vi "basic-lifetime-test.vi"(8 "error in (no error)":errorcluster) -> (0 "error out":errorcluster)   [LabVIEW 2021]
uses:
  <vilib>/addons/_JKI Toolkits/Caraya/classes/Test/Test.lvclass
  src/SMO/SMO.lvclass
  <vilib>/addons/_JKI Toolkits/Caraya/classes/Assert/Assert.lvclass
  src/SMO/Typedefs/SMOState --Enum.ctl
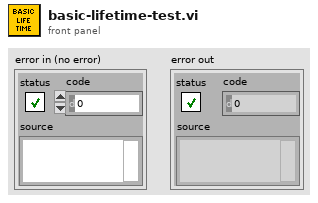
[diagram p1: front panel]
types:
  T1 = typedef "smo.lvlib/SMO.lvclass/SMOState --Enum.ctl" = enum16{"unknown", "Created", "Started", "Stopped"}
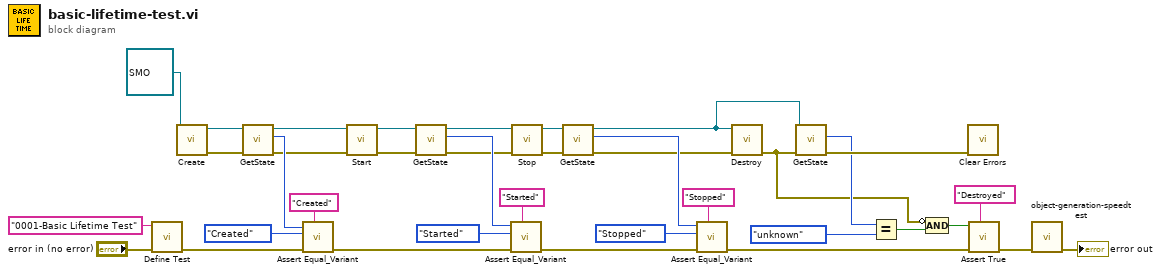
[diagram p0: block diagram]
diagram:
  n1 = call <vilib>:"Define Test.vi"("error in (no error)"="error in (no error)", "Label (VI Title)"="0001-Basic Lifetime Test") -> ("error out"=w33:errorcluster)  [unwired: 9 in]
  n2 = call "Create.vi"("SMO"=refnum<class "SMO.lvclass"> refnum ("Dependency Type")) -> ("error out"=w34:errorcluster, "SMO out"=w36:refnum<class "SMO.lvclass">)  [unwired: 8 in, 1 out]
  n3 = call "GetState.vi"("error in (no error)"=w34, "SMO"=w36) -> ("error out"=w29:errorcluster, "SMO State"=w32:T1, "SMO out"=w35:refnum<class "SMO.lvclass">)  [unwired: 7 in]
  n4 = call <vilib>:"Assert Equal_Variant.vi"("Label"="Created" ("Label (VI Title)"), "error in (no error)"=w33, "Y"=SMOState_--Enum."Created" ("SMO State"), "X"=w32) -> ("error out"=w25:errorcluster)  [unwired: 7 in]
  n5 = call "Start.vi"("error in (no error)"=w29, "SMO"=w35) -> ("error out"=w27:errorcluster, "SMO out"=w28:refnum<class "SMO.lvclass">)  [unwired: 8 in]
  n6 = call "GetState.vi"("error in (no error)"=w27, "SMO"=w28) -> ("error out"=w21:errorcluster, "SMO State"=w23:T1, "SMO out"=w22:refnum<class "SMO.lvclass">)  [unwired: 7 in]
  n7 = call <vilib>:"Assert Equal_Variant.vi"("Label"="Started" ("Label (VI Title)"), "error in (no error)"=w25, "Y"=SMOState_--Enum."Started" ("SMO State"), "X"=w23) -> ("error out"=w15:errorcluster)  [unwired: 7 in]
  n8 = call "Stop.vi"("error in (no error)"=w21, "SMO"=w22) -> ("error out"=w18:errorcluster, "SMO out"=w17:refnum<class "SMO.lvclass">)  [unwired: 8 in]
  n9 = call "GetState.vi"("error in (no error)"=w18, "SMO"=w17) -> ("error out"=w14:errorcluster, "SMO State"=w16:T1, "SMO out"=w13:refnum<class "SMO.lvclass">)  [unwired: 7 in]
  n10 = call <vilib>:"Assert Equal_Variant.vi"("Label"="Stopped" ("Label (VI Title)"), "error in (no error)"=w15, "Y"=SMOState_--Enum."Stopped" ("SMO State"), "X"=w16) -> ("error out"=w6:errorcluster)  [unwired: 7 in]
  n11 = call "Destroy.vi"("error in (no error)"=w14, "SMO"=w13) -> ("error out"=w7:errorcluster)  [unwired: 9 in]
  n12 = call "GetState.vi"("error in (no error)"=w7, "SMO"=w13) -> ("error out"=w11:errorcluster, "SMO State"=w9:T1)  [unwired: 7 in, 1 out]
  n13 = Equal?(x=w9, y=SMOState_--Enum."unknown" ("SMO State")) -> (x = y?=w8:bool)
  n14 = Compound Arithmetic op=AND(invert w7, w8) -> (w4:bool)
  n15 = call <vilib>:"Clear Errors.vi"("error in (no error)"=w11) -> ()  [unwired: 5 in, 2 out]
  n16 = call <vilib>:"Assert True.vi"("Label"="Destroyed" ("Label (VI Title)"), "error in (no error)"=w6, "True?"=w4) -> ("error out"=w3:errorcluster)  [unwired: 8 in]
  n17 = call "object-generation-speedtest.vi"("error in (no error)"=w3) -> ("error out"=→"error out":errorcluster)  [unwired: 10 in]
